vi "Demultiplexer_Laser80Calc160_AreaOut.vi"() -> ()   [LabVIEW 2012]
uses:
  <vilib>/Platform/TimedLoop/XDataNode/timing_clust.ctl
  <vilib>/Platform/TimedLoop/XDataNode/nitl_modes.ctl
  <vilib>/Platform/TimedLoop/XDataNode/wakeup.ctl
  <vilib>/rvi/Emulation/niFpgaSctlEmulationRegisterWithScheduler.vi
  <vilib>/rvi/eio/common/nirviEmuTemplateMethod_errors.vi
  <vilib>/rvi/Emulation/niFpgaSctlEmulationScheduler.vi
  <vilib>/rvi/FIFO/Fifo_Resource/nirvififoEmulationSetSize.vi
  <vilib>/rvi/DataTransferAndStorage/Container/Common/niFpgaContainerGetUniqueNameForEmu.vi
  <vilib>/rvi/eio/common/nirviEmuReportErrorAndStop.vi
  <vilib>/rvi/errors/niFpgaSetErrorForExecOnDevCompSimple.vi
  <vilib>/rvi/Emulation/niFpgaSctlEmulationFifoFullMgr.vi
  <vilib>/rvi/Emulation/niFpgaSctlEmulationResourceMgr.vi
  <vilib>/rvi/interface/RandomDataEmulation/niFpgaRandomDataHandleErrors.vi
  <vilib>/rvi/interface/RandomDataEmulation/nirviRandomDataFPGAFIFO.vi
  <vilib>/rvi/Emulation/niFpgaSctlEmulationGlobalWrite.vi
  <vilib>/Platform/TimedLoop/XDataNode/XDataNode.xnode
  <vilib>/eio/EIONode/EIONode.xnode
  <vilib>/rvi/DataTransferAndStorage/Container/XNode/niFpgaContainer.xnode
  <vilib>/rvi/FIFO/Fifo_Resource/nirvififoEmulationWrite.vi
  <vilib>/rvi/FIFO/Fifo_Resource/nirvififoEmulationRead.vi
  <vilib>/rvi/interface/RandomDataEmulation/nirviRandomDataFpgaReadWriteTemplate.vi
  <vilib>/rvi/FIFO/Fifo_Resource/nirvififoEmulationClear.vi
  <vilib>/Platform/TimedLoop/XDataNode/XDNodeRunTimeDep.lvlib
panel:
  in  "Switch for":i32=6 caption="Requested pixels"
  out "Laser pulse count A1":u16
  out "ToHost FIFO Overflow A2Ch2":bool
  out "ToHost FIFO Overflow A2Ch1":bool
  out "ToHost FIFO Overflow A1Ch2":bool
  in  "Samples per pixel Acq A2":u16=10000 caption="Samples per pixel Acq"
  in  "Samples per pixel Acq A1":u16=10000 caption="Samples per pixel Acq"
  in  "Requested pixels A2":u32=100000 caption="Requested pixels"
  in  "Samples per pixel A2":u16=10000 caption="Samples per pixel"
  out "ToHost FIFO Overflow A1Ch1":bool
  out "Acquiring":bool
  in  "Wait for trigger":bool
  in  "Acquire continuously":bool=TRUE
  in  "Requested pixels A1":u32=100000 caption="Requested pixels"
  in  "Clear Interloop FIFO":bool
  out "Interloop FIFO overflow":bool
  in  "Samples per pixel A1":u16=10000 caption="Samples per pixel"
  in  "Acquire":bool
  out "Interloop FIFO timeout":bool
  in  "Commit":bool
  out "Xpoint_Switch_Ready":bool
  in  "Xpoint_Switch_Write":bool
  in  "Clock Source":u8(ring)=3 items=["Tristate"=0, "Sync Clock (PXIe only)"=2, "Adapter Module Onboard Clock"=3, "Strobe from Crosspoint Switch"=4, "Strobe Bypass"=5]
  in  "Onboard_Clock_Write":bool
  in  "Onboard_Clock_Write_Data":u16
  out "Onboard_Clock_Ready":bool
  in  "Acq_Reset":bool
  # "6587 IO module configuration"
  # "Demultiplexer - Laser 80MHz/Calculate 160MHz\nArea as Ch1 output"
  # "Acquisition control"
  # "Area 1"
  # "Area 2"
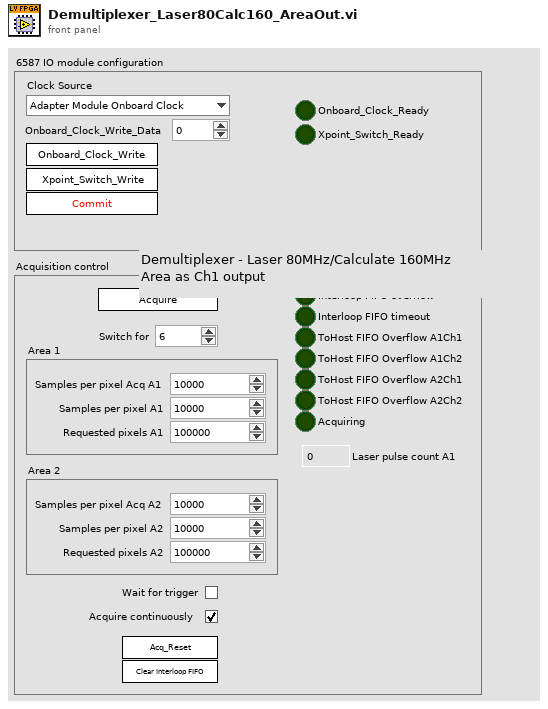
[diagram p1: front panel]
types:
  T1 = typedef "XDNodeRunTimeDep.lvlib/timing_clust.ctl" = cluster{"Expected End [f-1]":u64, "Actual End [f-1]":u64, "Finished Late? [f-1]":bool, "Expected End [i-1]":u64, "Actual End [i-1]":u64, "Finished Late? [i-1]":bool, "Expected Start [i]":u64, "Actual Start [i]":u64, "Expected Start [f]":u64, "Actual Start [f]":u64, "Source Name":string, "Structure Name":string, "Period":i64, "Deadline":i64, "Offset":i64, "Start":i64, "Priority":i32, "Timeout":i32, "Mode":T2, "Wakeup Reason":T3, "Error":errorcluster, "Source Type":string, "Secondary Source Type":string, "Global End Time":u64, "Global Start Time":u64, "Frame Duration":u64, "Iteration Duration":u64, "Assigned CPU":i32, "I/O Scan Engine Mode":u32}
  T2 = typedef "XDNodeRunTimeDep.lvlib/nitl_modes.ctl" = enum32{"No Change", "Process missed periods, maintain original phase", "Discard missed periods, maintain original phase", "Process missed periods, ignore original phase", "Discard missed periods, ignore original phase"}
  T3 = typedef "XDNodeRunTimeDep.lvlib/wakeup.ctl" = enum32{"Normal", "Aborted", "Asynchronous wakeup", "Timing source error", "Timed loop error", "Timeout"}
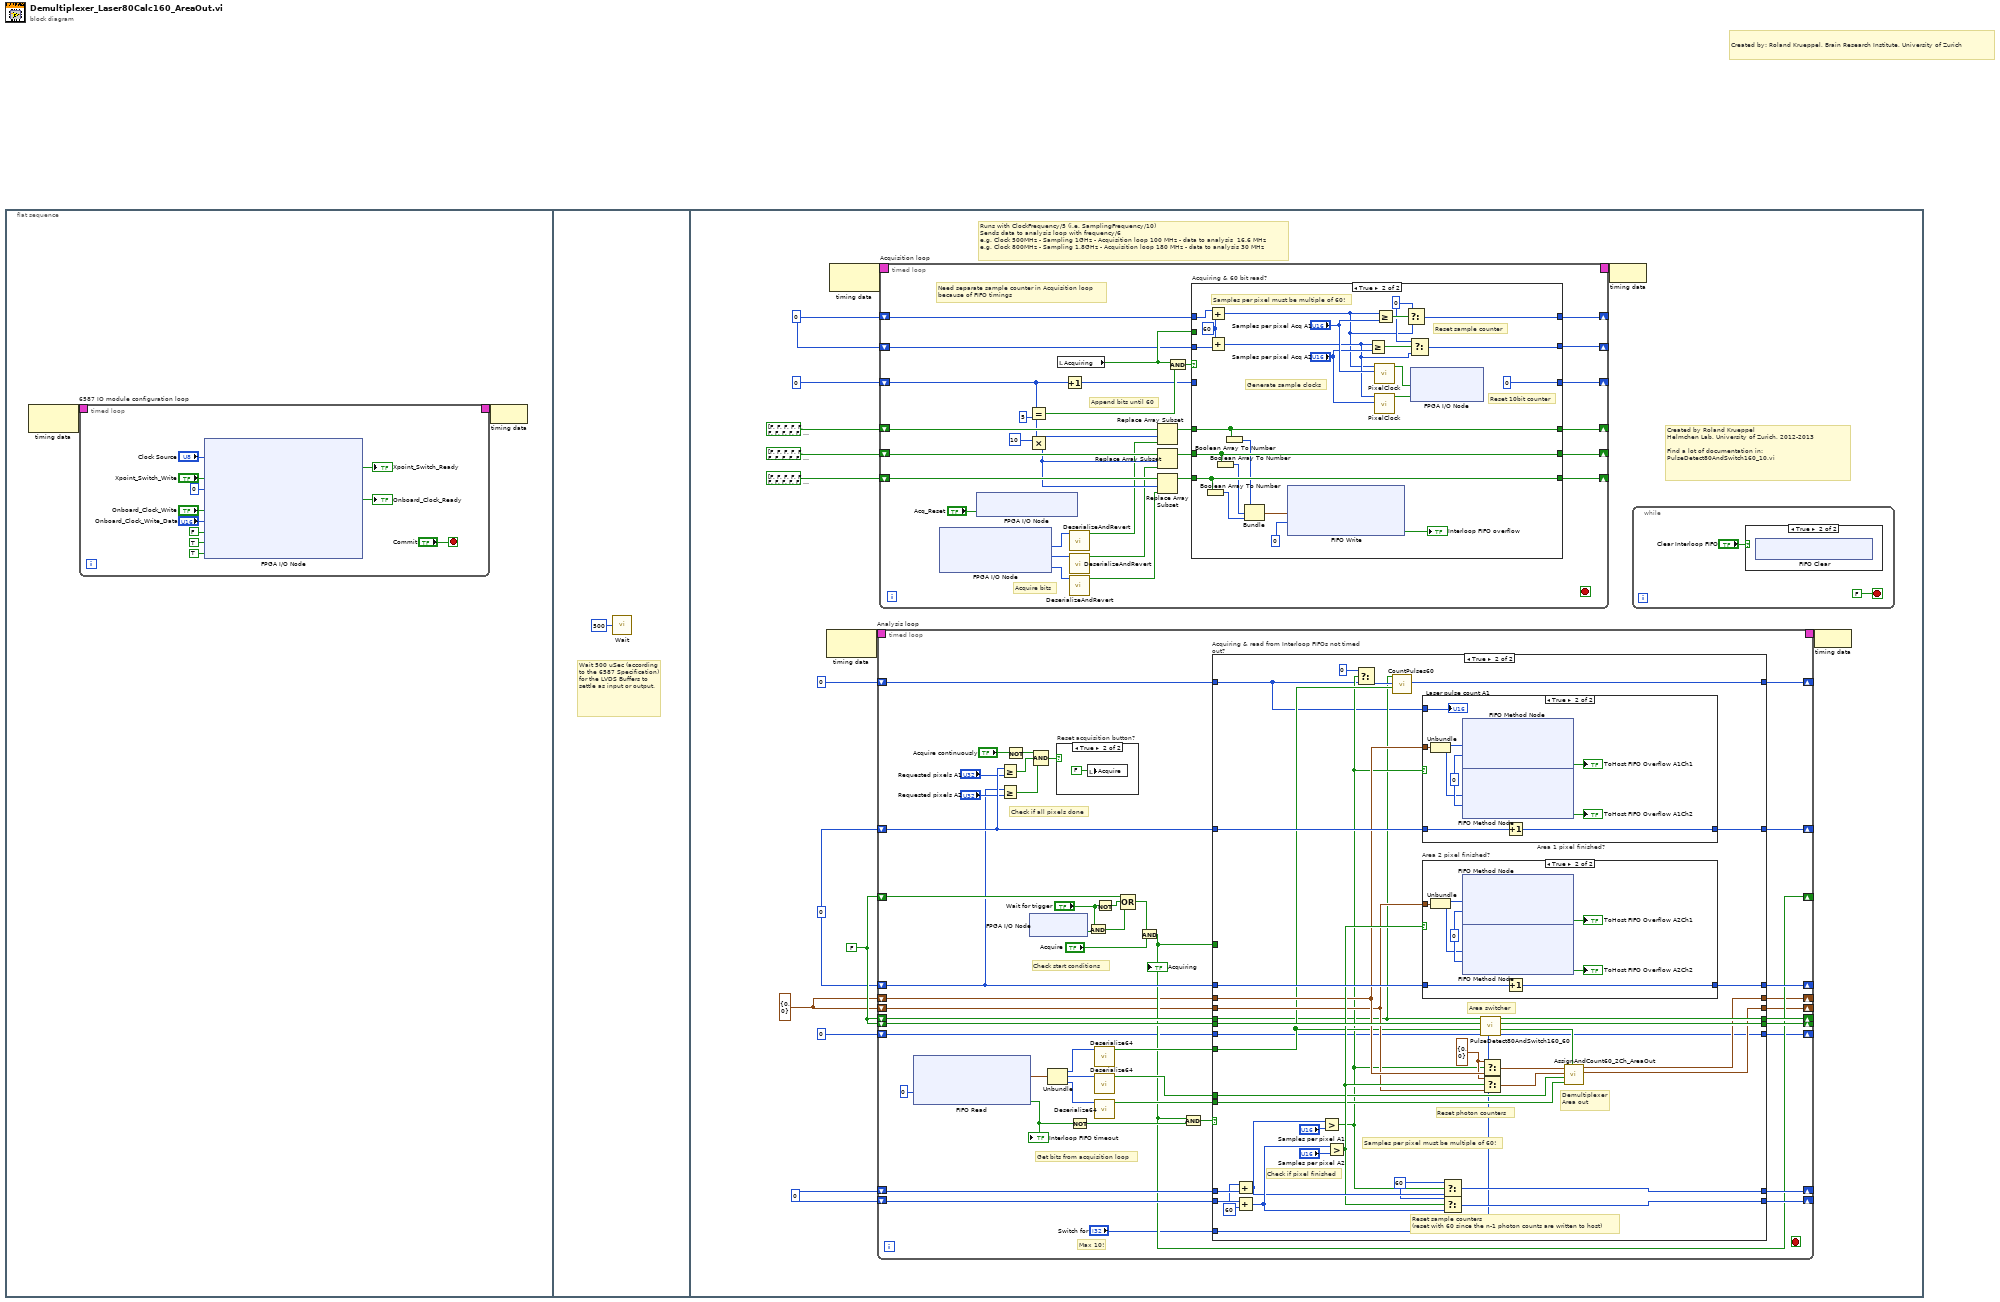
[diagram p0: block diagram]
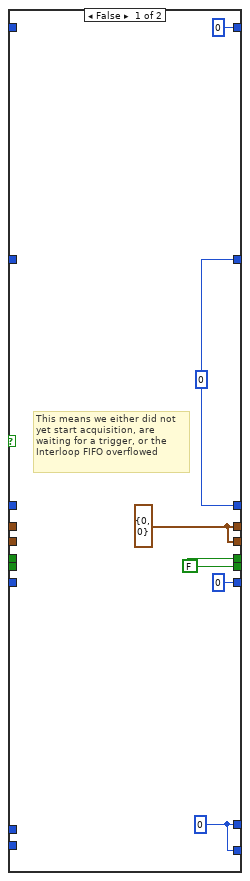
[diagram p5: hidden frame]
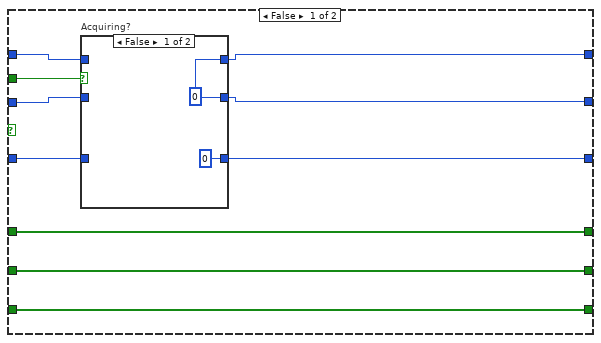
[diagram p8: hidden frame]
diagram:
  # "Created by: Roland Krueppel, Brain Research Institute, University of Zurich"
  n1 = flat-sequence {
    frame #0 {
      n2 = node-c288() -> (w2:T1)  [unwired: 1 in]
      n3 = timed-loop "6587 IO module configuration loop" {
        timing: w2 -> [_]
        timing-out: [_] -> w1
        stop <- "Commit" stop-if-true
        n4 = xnode "FPGA I/O Node"("IO Module\\Acq_IO_Clock_Source"="Clock Source", "IO Module\\Xpoint_Switch_Write"="Xpoint_Switch_Write", "IO Module\\LVDS_Data_Dir"=u16 0 ("IO Module\\LVDS_Data_Dir"), "IO Module\\Onboard_Clock_Write"="Onboard_Clock_Write", "IO Module\\Onboard_Clock_Write_Data"="Onboard_Clock_Write_Data", "IO Module\\SE_PFI0_WE"=FALSE ("IO Module\\SE_PFI0_WE"), "IO Module\\SE_PFI1_WE"=TRUE ("IO Module\\SE_PFI1_WE"), "IO Module\\SE_PFI2_WE"=TRUE ("IO Module\\SE_PFI2_WE")) -> ("IO Module\\Xpoint_Switch_Ready"=→"Xpoint_Switch_Ready":bool, "IO Module\\Onboard_Clock_Ready"=→"Onboard_Clock_Ready":bool)  [unwired: 10 in, 10 out]
      }
      n5 = node-c288(w1) -> ()
    }
    frame #1 {
      # "Wait 500 uSec (according to the 6587 Specification) for the LVDS Buffers to settle as input or output."
      n6 = call "Wait"("Count(uSec)"=u32 500) -> ()  [unwired: 1 out]
    }
    frame #2 {
      w22 = cluster{u16, u16} {0, 0} ("output cluster")
      w23 = u16 0
      w21 = u32 0 ("Cycle counter out")
      w24 = u16 0
      w25 = FALSE ("Last laser bit out")
      # "Runs with ClockFrequency/5 (i.e. SamplingFrequency/10)\nSends data to analysis loop with frequency/6\ne.g. Clock 500MHz - Sampling 1GHz - Acquisition loop 100 MHz - data to analysis  16.6 MHz\ne.g. Clock 800MHz - Sampling 1.8GHz - Acquisition loop 180 MHz - data to analysis 30 MHz"
      # "Created by Roland Krueppel\nHelmchen Lab, University of Zurich, 2012-2013\n\nFind a lot of documentation in:\nPulseDetect80AndSwitch160_10.vi"
      n7 = node-c288() -> (w31:T1)  [unwired: 1 in]
      n8 = node-c288() -> (w33:T1)  [unwired: 1 in]
      n9 = timed-loop "Analysis loop" {
        timing: w31 -> [_]
        timing-out: [_] -> w30
        shift-right: [w79] -> _
        shift-left: w25 -> [w82]
        shift-right: [w81] -> _
        shift-left: w25 -> [w80]
        shift-right: [w55] -> _
        shift-left: w24 -> [w78]
        shift-right: [w53] -> _
        shift-left: w21 -> [w77]
        shift-right: [w51] -> _
        shift-left: w25 -> [w66]
        shift-right: [w54] -> _
        shift-left: w24 -> [w61]
        shift-right: [w52] -> _
        shift-left: w21 -> [w59]
        shift-right: [w42] -> _
        shift-left: w22 -> [w44]
        shift-right: [w41] -> _
        shift-left: w22 -> [w43]
        shift-right: [w40] -> _
        shift-left: u16 0 ("New pulse count") -> [w39]
        shift-right: [w38] -> _
        shift-left: 0 ("Fill after last") -> [w37]
        stop <- _ stop-if-true
        # "Max 10!"
        # "Get bits from acquisition loop"
        # "Check start conditions"
        # "Check if all pixels done"
        n10 = xnode ("FIFO Read")("Timeout"=0) -> ("Element"=w48:cluster{"Laser":u64, "Ch0":u64, "Ch1":u64}, "Timed Out?"=w49:bool)  [unwired: 1 in, 1 out]
        "Interloop FIFO timeout" <- w49
        n11 = Greater Or Equal?(x=w77, y="Requested pixels A1") -> (x >= y?=w57:bool)
        n12 = Greater Or Equal?(x=w59, y="Requested pixels A2") -> (x >= y?=w56:bool)
        n13 = Not(x="Acquire continuously") -> (.not. x?=w58:bool)
        n14 = xnode "FPGA I/O Node"() -> ("TriggerIn"=w72:bool)  [unwired: 1 in, 1 out]
        n15 = Compound Arithmetic op=AND(w58, w57, w56) -> (w74:bool)
        n16 = Unbundle(w48) -> ("Laser"=w47:u64, "Ch0"=w46:u64, "Ch1"=w45:u64)
        n17 = case "Reset acquisition button?" shown="True" w74 {
          frame False {
          }
          frame True {
            n18 = local write "Acquire"(FALSE ("Acquire")) -> ()
          }
        }
        n19 = Not(x=w49) -> (.not. x?=w67:bool)
        n20 = And(x="Wait for trigger", y=w72) -> (x .and. y?=w69:bool)
        n21 = call "Deserialize64.vi"("U64 input"=w47) -> ("60bit output"=w64:bool[])  [unwired: 10 in]
        n22 = call "Deserialize64.vi"("U64 input"=w46) -> ("60bit output"=w63:bool[])  [unwired: 10 in]
        n23 = call "Deserialize64.vi"("U64 input"=w45) -> ("60bit output"=w62:bool[])  [unwired: 10 in]
        n24 = Not(x="Wait for trigger") -> (.not. x?=w70:bool)
        n25 = Compound Arithmetic op=OR(w66, w70, w69) -> (w68:bool)
        n26 = And(x=w68, y="Acquire") -> (x .and. y?=w51:bool)
        "Acquiring" <- w51
        n27 = And(x=w51, y=w67) -> (x .and. y?=w65:bool)
        n28 = case "Acquiring & read from Interloop FIFOs not timed out?" shown="True" w65 {
          tunnel: w82 -> [w99 w144]
          tunnel: w44 -> [w103 w140]
          tunnel: [w98 w143] -> w81
          tunnel: w80 -> [w100 w125]
          tunnel: [w97 w142] -> w79
          tunnel: w78 -> [w102 w158]
          tunnel: w77 -> [w101 w154]
          tunnel: w64 -> [_ w130]
          tunnel: w63 -> [_ w135]
          tunnel: w51 -> [w104 _]
          tunnel: w62 -> [_ w134]
          tunnel: w61 -> [w91 w156]
          tunnel: w59 -> [w94 w153]
          tunnel: [w92 w146] -> w55
          tunnel: [w90 w148] -> w54
          tunnel: [w96 w132] -> w42
          tunnel: [w95 w151] -> w53
          tunnel: [w93 w152] -> w52
          tunnel: w43 -> [w89 w137]
          tunnel: [w88 w131] -> w41
          tunnel: [w86 w129] -> w40
          tunnel: w39 -> [w87 w124]
          tunnel: [w84 w123] -> w38
          tunnel: w37 -> [w85 w122]
          tunnel: "Switch for" -> [_ w121]
          frame False {
            n29 = case "Acquiring?" shown="True" w104 {
              tunnel: w103 -> [_ w118]
              tunnel: w102 -> [_ w115]
              tunnel: w101 -> [_ w117]
              tunnel: w100 -> [_ w120]
              tunnel: w99 -> [_ w119]
              tunnel: [w110 w120] -> w98
              tunnel: [w110 w119] -> w97
              tunnel: [w108 w118] -> w96
              tunnel: [w109 w117] -> w95
              tunnel: w94 -> [_ w116]
              tunnel: [w109 w116] -> w93
              tunnel: [w107 w115] -> w92
              tunnel: [w107 w114] -> w90
              tunnel: w91 -> [_ w114]
              tunnel: w89 -> [_ w113]
              tunnel: [w108 w113] -> w88
              tunnel: w87 -> [_ w112]
              tunnel: [u16 0 ("New pulse count") w112] -> w86
              tunnel: w85 -> [_ w111]
              tunnel: [0 ("Fill after last") w111] -> w84
              frame False {
                w108 = cluster{u16, u16} {0, 0} ("output cluster")
                w109 = u32 0 ("Cycle counter out")
                w107 = u16 0
                w110 = FALSE ("Last laser bit out")
                # "This means we either did not\nyet start acquisition, are\nwaiting for a trigger, or the\nInterloop FIFO overflowed"
              }
              frame True {
                # "This means we are\nreading faster here\nthan acquiring in\nAcquisition loop\n-> keep all values"
              }
            }
          }
          frame True {
            w133 = cluster{u16, u16} {0, 0} ("t")
            w145 = u16 60 ("t")
            w155 = u16 60
            # "Samples per pixel must be multiple of 60!"
            # "Demultiplexer\nArea out"
            # "Reset photon counters"
            # "Area switcher"
            # "Check if pixel finished"
            # "Reset sample counters\n(reset with 60 since the n-1 photon counts are written to host)"
            n30 = Add(x=w155, y=w158) -> (x+y=w147:u16)
            n31 = Add(x=w156, y=w155) -> (x+y=w149:u16)
            n32 = Greater?(x=w147, y="Samples per pixel A1") -> (0:w128:bool)
            n33 = Greater?(x=w149, y="Samples per pixel A2") -> (0:w141:bool)
            n34 = Select(t=u16 0, s=w128, f=w124) -> (s? t:f=w127:u16)
            n35 = call "CountPulses60.vi"("60bit input"=w130, "Previous pulse count"=w127, "Last sample"=w125) -> ("New pulse count"=w129:u16)  [unwired: 7 in, 1 out]
            n36 = case "Area 1 pixel finished?" shown="True" w128 {
              tunnel: w140 -> [_ w172]
              tunnel: w154 -> [w168 w176]
              tunnel: [w168 w175] -> w151
              tunnel: w124 -> [_ w169]
              frame False {
              }
              frame True {
                w177 = 0 ("Timeout")
                n37 = Unbundle(w172) -> (w171:u16, w170:u16)
                n38 = xnode ("FIFO Method Node")("Element"=w171, "Timeout"=w177) -> ("Timed Out?"=→"ToHost FIFO Overflow A1Ch1":bool)  [unwired: 1 in, 1 out]
                n39 = xnode ("FIFO Method Node")("Element"=w170, "Timeout"=w177) -> ("Timed Out?"=→"ToHost FIFO Overflow A1Ch2":bool)  [unwired: 1 in, 1 out]
                n40 = Increment(x=w176) -> (x+1=w175:u32)
                "Laser pulse count A1" <- w169
              }
            }
            n41 = case "Area 2 pixel finished?" shown="True" w141 {
              tunnel: w153 -> [w159 w166]
              tunnel: [w159 w165] -> w152
              tunnel: w137 -> [_ w162]
              frame False {
              }
              frame True {
                w167 = 0 ("Timeout")
                n42 = Unbundle(w162) -> (w161:u16, w160:u16)
                n43 = xnode ("FIFO Method Node")("Element"=w161, "Timeout"=w167) -> ("Timed Out?"=→"ToHost FIFO Overflow A2Ch1":bool)  [unwired: 1 in, 1 out]
                n44 = xnode ("FIFO Method Node")("Element"=w160, "Timeout"=w167) -> ("Timed Out?"=→"ToHost FIFO Overflow A2Ch2":bool)  [unwired: 1 in, 1 out]
                n45 = Increment(x=w166) -> (x+1=w165:u32)
              }
            }
            n46 = Select(t=w145, s=w128, f=w147) -> (s? t:f=w146:u16)
            n47 = Select(t=w145, s=w141, f=w149) -> (s? t:f=w148:u16)
            n48 = call "PulseDetect80AndSwitch160_60.vi"("Switch for"=w121, "Fill from last"=w122, "Laser bits in"=w130, "Last area in"=w144, "Last laser bit in"=w125) -> ("Fill after last"=w123:i32, "Area bits out"=w139:bool[], "New last area out"=w142:bool, "New last laser bit out"=w143:bool)  [unwired: 3 in]
            n49 = Select(t=w133, s=w128, f=w140) -> (s? t:f=w138:cluster{u16, u16})
            n50 = Select(t=w133, s=w141, f=w137) -> (s? t:f=w136:cluster{u16, u16})
            n51 = call "AssignAndCount60_2Ch_AreaOut.vi"("Area bits in"=w139, "PMT bits Ch2 in"=w134, "PMT bits Ch1 in"=w135, "Photon counters area 2 in"=w136, "Photon counters area 1 in"=w138) -> ("Photon counters area 2 out"=w131:cluster{u16, u16}, "Photon counters area 1 out"=w132:cluster{u16, u16})  [unwired: 5 in]
          }
        }
      }
      n52 = timed-loop "Acquisition loop" {
        timing: w33 -> [_]
        timing-out: [_] -> w32
        shift-right: [w201] -> _
        shift-left: bool[] [FALSE, FALSE, FALSE, FALSE, FALSE, FALSE, FALSE, FALSE, FALSE, FALSE, FALSE, FALSE, FALSE, FALSE, FALSE, FALSE, FALSE, FALSE, FALSE, FALSE, FALSE, FALSE, FALSE, FALSE, FALSE, FALSE, FALSE, FALSE, FALSE, FALSE, FALSE, FALSE, FALSE, FALSE, FALSE, FALSE, FALSE, FALSE, FALSE, FALSE, FALSE, FALSE, FALSE, FALSE, FALSE, FALSE, FALSE, FALSE, FALSE, FALSE, FALSE, FALSE, FALSE, FALSE, FALSE, FALSE, FALSE, FALSE, FALSE, FALSE, FALSE, FALSE, FALSE, FALSE] ("Boolean array") -> [w209]
        shift-right: [w200] -> _
        shift-left: bool[] [FALSE, FALSE, FALSE, FALSE, FALSE, FALSE, FALSE, FALSE, FALSE, FALSE, FALSE, FALSE, FALSE, FALSE, FALSE, FALSE, FALSE, FALSE, FALSE, FALSE, FALSE, FALSE, FALSE, FALSE, FALSE, FALSE, FALSE, FALSE, FALSE, FALSE, FALSE, FALSE, FALSE, FALSE, FALSE, FALSE, FALSE, FALSE, FALSE, FALSE, FALSE, FALSE, FALSE, FALSE, FALSE, FALSE, FALSE, FALSE, FALSE, FALSE, FALSE, FALSE, FALSE, FALSE, FALSE, FALSE, FALSE, FALSE, FALSE, FALSE, FALSE, FALSE, FALSE, FALSE] ("Boolean array") -> [w208]
        shift-right: [w199] -> _
        shift-left: 0 -> [w198]
        shift-right: [w194] -> _
        shift-left: bool[] [FALSE, FALSE, FALSE, FALSE, FALSE, FALSE, FALSE, FALSE, FALSE, FALSE, FALSE, FALSE, FALSE, FALSE, FALSE, FALSE, FALSE, FALSE, FALSE, FALSE, FALSE, FALSE, FALSE, FALSE, FALSE, FALSE, FALSE, FALSE, FALSE, FALSE, FALSE, FALSE, FALSE, FALSE, FALSE, FALSE, FALSE, FALSE, FALSE, FALSE, FALSE, FALSE, FALSE, FALSE, FALSE, FALSE, FALSE, FALSE, FALSE, FALSE, FALSE, FALSE, FALSE, FALSE, FALSE, FALSE, FALSE, FALSE, FALSE, FALSE, FALSE, FALSE, FALSE, FALSE] ("Boolean array") -> [w197]
        shift-right: [w193] -> _
        shift-left: w23 -> [w183]
        shift-right: [w192] -> _
        shift-left: w23 -> [w182]
        stop <- _ stop-if-true
        # "Need separate sample counter in Acquisition loop\nbecause of FIFO timings"
        # "Append bits until 60"
        # "Acquire bits"
        n53 = xnode "FPGA I/O Node"() -> ("IO Module\\LVDS_Ch0_Rd"=w189:u16, "IO Module\\LVDS_Ch1_Rd"=w187:u16, "IO Module\\LVDS_Ch2_Rd"=w185:u16)  [unwired: 3 in, 3 out]
        n54 = xnode "FPGA I/O Node"("IO Module\\Acq_Reset"="Acq_Reset") -> ()  [unwired: 1 in, 1 out]
        n55 = Equal?(x=w198, y=5) -> (x = y?=w205:bool)
        n56 = Multiply(x=10 ("y"), y=w198) -> (x*y=w196:i32)
        n57 = local read "Acquiring"() -> (w191:bool)
        n58 = Increment(x=w198) -> (x+1=w190:i32)
        n59 = call "DeserializeAndRevert.vi"("U16 input"=w189) -> ("10bit output"=w188:bool[])  [unwired: 10 in]
        n60 = call "DeserializeAndRevert.vi"("U16 input"=w187) -> ("10bit output"=w186:bool[])  [unwired: 10 in]
        n61 = call "DeserializeAndRevert.vi"("U16 input"=w185) -> ("10bit output"=w184:bool[])  [unwired: 10 in]
        n62 = Replace Array Subset(array=w209, new element=w188, index=w196) -> (w203:bool[])
        n63 = Replace Array Subset(array=w208, new element=w186, index=w196) -> (w202:bool[])
        n64 = Replace Array Subset(array=w197, new element=w184, index=w196) -> (w195:bool[])
        n65 = And(x=w191, y=w205) -> (x .and. y?=w204:bool)
        n66 = case "Acquiring & 60 bit read?" shown="True" w204 {
          tunnel: w203 -> [w220 w246]
          tunnel: w202 -> [w219 w248]
          tunnel: [w220 w246] -> w201
          tunnel: [w219 w248] -> w200
          tunnel: [w213 0] -> w199
          tunnel: w190 -> [w214 _]
          tunnel: w195 -> [w218 w247]
          tunnel: [w218 w247] -> w194
          tunnel: w183 -> [w216 w228]
          tunnel: [w211 w244] -> w193
          tunnel: w182 -> [w215 w230]
          tunnel: [w212 w239] -> w192
          tunnel: w191 -> [w217 _]
          frame False {
            n67 = case "Acquiring?" shown="False" w217 {
              tunnel: w216 -> [_ w225]
              tunnel: w215 -> [_ w224]
              tunnel: w214 -> [_ w223]
              tunnel: [w222 w225] -> w211
              tunnel: [w222 w224] -> w212
              tunnel: [0 w223] -> w213
              frame False {
                w222 = u16 0
              }
              frame True {
              }
            }
          }
          frame True {
            w226 = u16 60 ("y")
            w240 = u16 0 ("t")
            # "Reset 10bit counter"
            # "Reset sample counter"
            # "Samples per pixel must be multiple of 60!"
            # "Generate sample clocks"
            n68 = Boolean Array To Number(Boolean array=w247) -> (number=w234:u64)
            n69 = Add(x=w228, y=w226) -> (x+y=w227:u16)
            n70 = Add(x=w226, y=w230) -> (x+y=w229:u16)
            n71 = Boolean Array To Number(Boolean array=w248) -> (number=w235:u64)
            n72 = Boolean Array To Number(Boolean array=w246) -> (number=w236:u64)
            n73 = Bundle(w236, w235, w234) -> (w233:cluster{u64, u64, u64})  [unwired: 1 in]
            n74 = xnode ("FIFO Write")("Element"=w233, "Timeout"=0) -> ("Timed Out?"=→"Interloop FIFO overflow":bool)  [unwired: 1 in, 1 out]
            n75 = Greater Or Equal?(x=w229, y="Samples per pixel Acq A2") -> (x >= y?=w241:bool)
            n76 = call "PixelClock.vi"("Samples per pixel"="Samples per pixel Acq A1", "Sample counter"=w227) -> ("Pixel clock"=w242:bool)  [unwired: 9 in]
            n77 = call "PixelClock.vi"("Samples per pixel"="Samples per pixel Acq A2", "Sample counter"=w229) -> ("Pixel clock"=w237:bool)  [unwired: 9 in]
            n78 = Greater Or Equal?(x=w227, y="Samples per pixel Acq A1") -> (x >= y?=w245:bool)
            n79 = Select(t=w240, s=w245, f=w227) -> (s? t:f=w244:u16)
            n80 = Select(t=w240, s=w241, f=w229) -> (s? t:f=w239:u16)
            n81 = xnode "FPGA I/O Node"("Pixel clock A1"=w242, "Pixel clock A2"=w237) -> ()  [unwired: 2 in, 2 out]
          }
        }
      }
      n82 = node-c288(w32) -> ()
      n83 = while {
        stop <- FALSE stop-if-true
        n84 = case shown="True" "Clear Interloop FIFO" {
          frame False {
          }
          frame True {
            n85 = xnode ("FIFO Clear")() -> ()  [unwired: 1 in, 1 out]
          }
        }
      }
      n86 = node-c288(w30) -> ()
    }
  }
